vi "Add Port Outgoing Section.vi"(7 "highlight?":bool, 8 "error in":errorcluster, 11 "ports ref":T1 format="%.0x") -> (0 "error out":errorcluster, 2 "port outgoing ref out":T1=18446744073709551615 format="%.0x", 3 "ports ref out":T1 format="%.0x")   [LabVIEW 2020, in "AIM ARINC 664 Scripting.lvlib"]
doc: "Add the Outgoing Port page to the system definion.."
uses:
  AIM ARINC 664 Scripting.lvlib
  <vilib>/NI VeriStand/Custom Device API/Custom Device Item Ref.ctl
  Constants.vi
  <vilib>/NI VeriStand/Custom Device API/Custom Device API.lvlib
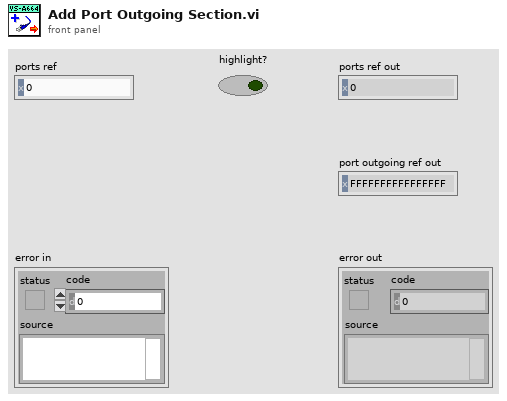
[diagram p1: front panel]
types:
  T1 = typedef "Custom Device API.lvlib/Custom Device Item Ref.ctl" = u64
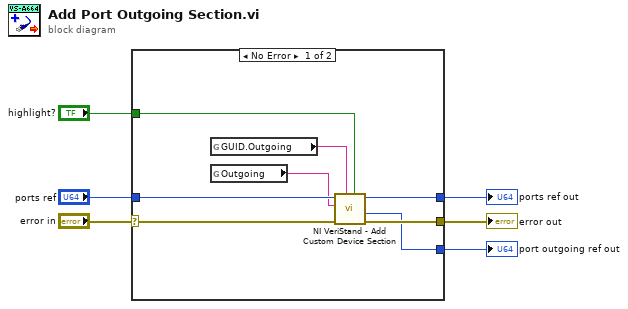
[diagram p0: block diagram]
diagram:
  n1 = case shown="No Error" "error in" {
    selector: "error in" -> [w11 w16]
    tunnel: "highlight?" -> [w13 _]
    tunnel: "ports ref" -> [w12 w15]
    tunnel: [w10 w16] -> w4
    tunnel: [w8 w15] -> w3
    tunnel: [w7 _] -> w1
    frame No Error {
      n2 = global read "Constants.vi" "GUID.Outgoing"() -> (w14:string)
      n3 = global read "Constants.vi" "Outgoing"() -> (w9:string)
      n4 = call <vilib>:"NI VeriStand - Add Custom Device Section.vi"("Highlight? (F)"=w13, "GUID (Default Section)"=w14, "error in (no error)"=w11, "Section Name"=w9, "Parent Ref in"=w12) -> ("error out"=w10:errorcluster, "Section Ptr"=w7:T1, "Parent Ref out"=w8:T1)  [unwired: 3 in, 1 out]
    }
    frame Error {
    }
  }
  "error out" <- w4
  "ports ref out" <- w3
  "port outgoing ref out" <- w1
